vi "__main.vi"(8 "error in (no error)":errorcluster, 10 "udpCxcn":refnum<k16>, 11 "BME280 in":refnum<class "BME280.lvclass">) -> (0 "error out":errorcluster, 3 "BME280 out":refnum<class "BME280.lvclass">)   [LabVIEW 2020, in "BME280.lvclass"]
uses:
  BME280.lvclass
  BME280.lvclass/BME280.ctl
  Single Weather.ctl
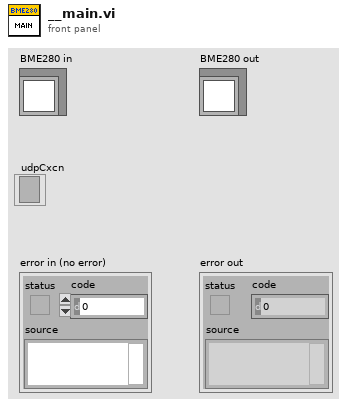
[diagram p1: front panel]
types:
  T1 = typedef "BME280.lvclass/Single Weather.ctl" = cluster{"temperature":dbl, "humidity":dbl, "pressure":dbl}
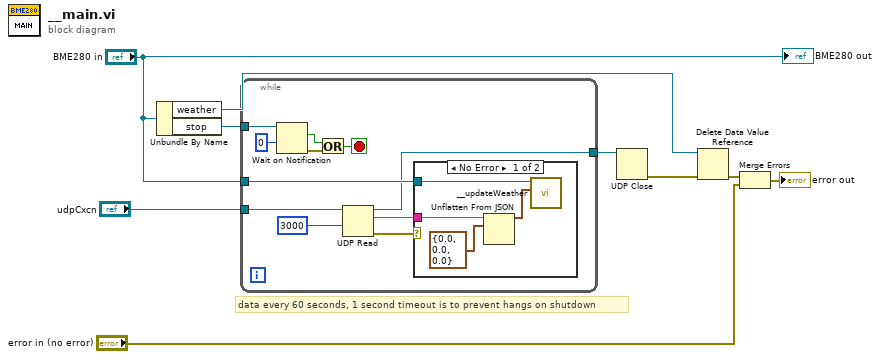
[diagram p0: block diagram]
diagram:
  # "data every 60 seconds, 1 second timeout is to prevent hangs on shutdown"
  n1 = Unbundle By Name("BME280 in") -> ("weather"=w6:refnum<data-value>, "stop"=w9:refnum<notifier>)
  n2 = while {
    tunnel: w9 -> [w20]
    tunnel: "udpCxcn" -> [w10]
    tunnel: "BME280 in" -> [w14]
    tunnel: [w13] -> w8
    stop <- w16 stop-if-true
    n3 = Wait on Notification(notifier=w20, timeout in ms (-1)=0) -> (notification=w17:bool, error out=w18:errorcluster)  [unwired: 2 in, 2 out]
    n4 = Or(x=w17, y=w18) -> (x .or. y?=w16:bool)
    n5 = UDP Read(connection ID=w10, timeout ms (25000)=3000) -> (data out=w15:string, error out=w11:errorcluster, 3:w13:refnum<k16>)  [unwired: 2 in, 2 out]
    n6 = case shown="No Error" w11 {
      tunnel: w15 -> [w24 _]
      tunnel: w14 -> [w22 _]
      frame No Error {
        n7 = Unflatten From JSON(JSON string=w24, type and defaults=T1 {"temperature"=0.0, "humidity"=0.0, "pressure"=0.0} ("singleWeather")) -> (value=w21:T1)  [unwired: 5 in, 1 out]
        n8 = call "__updateWeather.vi"("singleWeather"=w21, "BME280 in"=w22) -> ()  [unwired: 9 in, 1 out]
      }
      frame Error {
      }
    }
  }
  n9 = UDP Close(connection ID=w8) -> (error out=w7:errorcluster)  [unwired: 1 in, 1 out]
  n10 = Delete Data Value Reference(data value reference=w6, error in=w7) -> (error out=w4:errorcluster)  [unwired: 1 out]
  n11 = Merge Errors(w4, "error in (no error)") -> (→"error out":errorcluster)
  "BME280 out" <- "BME280 in"
